vi "Get UIAs prefixes.vi"(11 "DualScreen in":refnum<class "DualScreen.lvclass">) -> (2 "2nd UIA prefix":string, 3 "1st UIA prefix":string)   [LabVIEW 2020, in "DualScreen.lvlib" / "DualScreen.lvclass"]
uses:
  DualScreen.lvclass
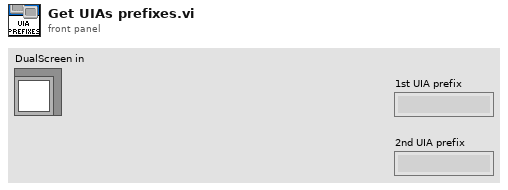
[diagram p1: front panel]
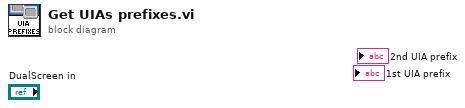
[diagram p0: block diagram]
diagram:
